vi "Data Viewer.vi"(8 "error in (no error)":errorcluster, 10 "Starting Waveforms":waveform(dbl)[](array[waveform])) -> (0 "error out":errorcluster, 3 "Data Viewer out":refnum<class "Data Viewer.lvclass">)   [LabVIEW 2020, in "2. Basic Panel Actors.lvlib" / "Data Viewer.lvclass"]
doc: "Initializes the Data Viewer Panel Actor.\n----\nCopyright: MGI 2017\nAuthor: Derek Trepanier"
uses:
  Data Viewer.lvclass
  Data Viewer.lvclass/Data Viewer.ctl
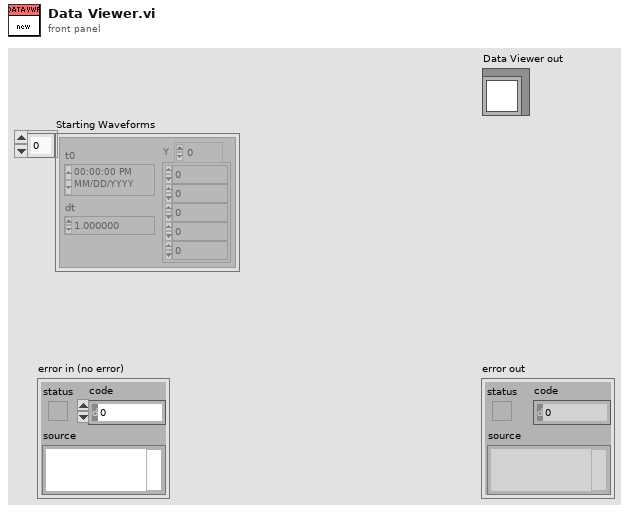
[diagram p1: front panel]
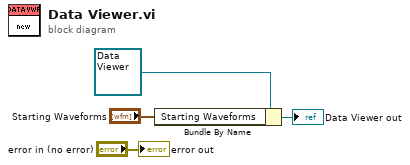
[diagram p0: block diagram]
diagram:
  n1 = Bundle By Name(cluster=refnum<class "Data Viewer.lvclass"> refnum ("Data Viewer in"), "Starting Waveforms"="Starting Waveforms") -> (→"Data Viewer out":refnum<class "Data Viewer.lvclass">)
  "error out" <- "error in (no error)"
